vi "Test_GetChannelsList.vi"() -> ()   [LabVIEW 2019]
uses:
  ByteQXAPIBase/ByteQXAPIBase.lvclass
panel:
  out "test passed?":bool
  out "error out":errorcluster
  out "channels":string[](array[string])
  in  "asset code":string
  in  "Auth token":string
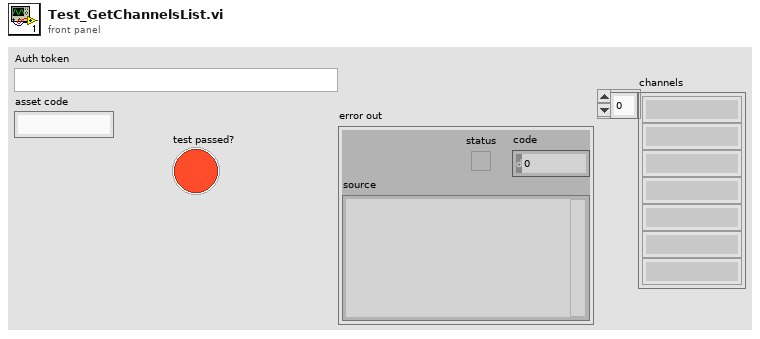
[diagram p1: front panel]
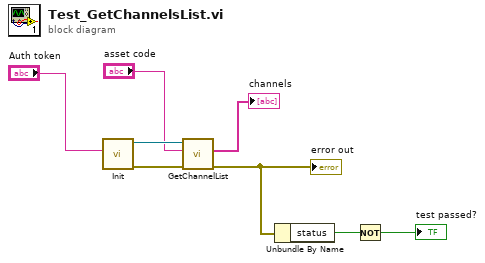
[diagram p0: block diagram]
diagram:
  n1 = call "Init.vi"("Auth token"="Auth token") -> ("error out"=w7:errorcluster, "ByteQXAPIBase out"=w8:refnum<class "ByteQXAPIBase.lvclass">)  [unwired: 9 in]
  n2 = call "GetChannelList.vi"("error in (no error)"=w7, "asset code"="asset code", "ByteGSAPIBase in"=w8) -> ("error out"=w3:errorcluster, "channels"=→"channels":string[])  [unwired: 6 in, 1 out]
  "error out" <- w3
  n3 = Unbundle By Name(w3) -> ("status"=w2:bool)
  n4 = Not(x=w2) -> (.not. x?=→"test passed?":bool)
